vi "3Pixel.vi"() -> (3 "3 pixel":u32)   [LabVIEW 2009, in "menu item.lvclass"]
uses:
  menu item.lvclass
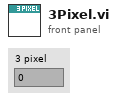
[diagram p1: front panel]
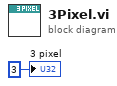
[diagram p0: block diagram]
diagram:
  "3 pixel" <- u32 3 ("1 pixel")
